vi "Get_Word_JSON.vi"(7 "API Key":string, 8 "error in (no error)":errorcluster, 10 "Word":string, 11 "client handle":T1) -> (0 "error out":errorcluster, 1 "Valid Definition?":bool, 2 "body":string, 3 "client handle out":T1)   [LabVIEW 2018, in "MerriamWebsterJSON.lvlib"]
uses:
  MerriamWebsterJSON.lvlib
  <vilib>/httpClient/ClientHandle.ctl
  <vilib>/httpClient/LabVIEWHTTPClient.lvlib
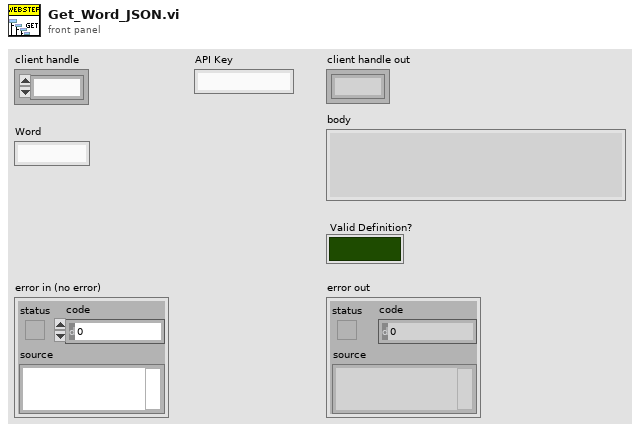
[diagram p1: front panel]
types:
  T1 = typedef "LabVIEWHTTPClient.lvlib/ClientHandle.ctl" = refnum<k1>
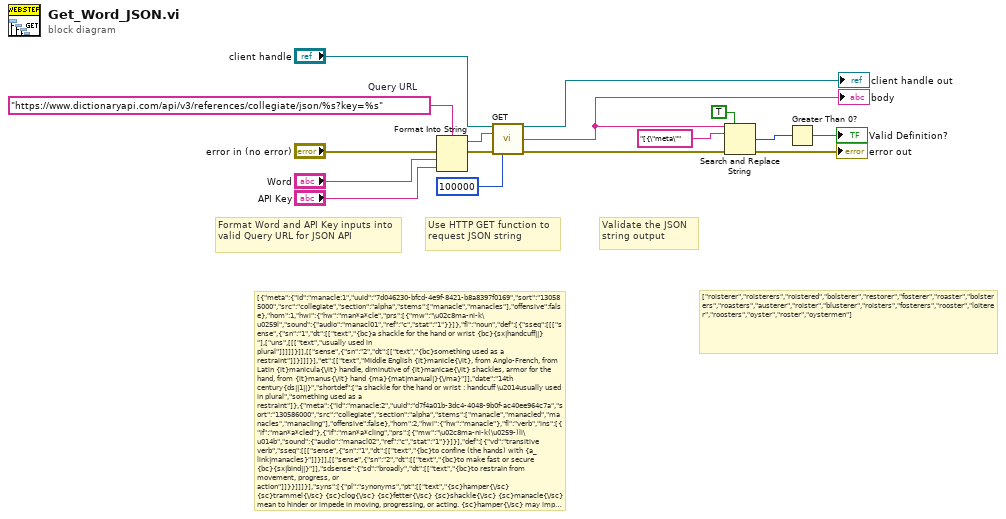
[diagram p0: block diagram]
diagram:
  w14 = "https://www.dictionaryapi.com/api/v3/references/collegiate/json/%s?key=%s"  # Query URL
  # "[{\"meta\":{\"id\":\"manacle:1\",\"uuid\":\"7d046230-bfcd-4e9f-8421-b8a8397f0169\",\"sort\":\"130585000\",\"src\":\"collegiate\",\"section\":\"alpha\",\"stems\":[\"manacle\",\"manacles\"],\"offensive\":false},\"hom\":1,\"hwi\":{\"hw\":\"man*a*cle\",\"prs\":[{\"mw\":\"\\u02c8ma-ni-k\\u0259l\",\"sound\":{\"audio\":\"manacl01\",\"ref\":\"c\",\"stat\":\"1\"}}]},\"fl\":\"noun\",\"def\":[{\"sseq\":[[[\"sense\",{\"sn\":\"1\",\"dt\":[[\"text\",\"{bc}a shackle for the hand or wrist {bc}{sx|handcuff||} \"],[\"uns\",[[[\"text\",\"usually used in plural\"]]]]]}]],[[\"sense\",{\"sn\":\"2\",\"dt\":[[\"text\",\"{bc}something used as a restraint\"]]}]]]}],\"et\":[[\"text\",\"Middle English {it}manicle{\\/it}, from Anglo-French, from Latin {it}manicula{\\/it} handle, diminutive of {it}manicae{\\/it} shackles, armor for the hand, from {it}manus{\\/it} hand {ma}{mat|manual|}{\\/ma}\"]],\"date\":\"14th century{ds||1||}\",\"shortdef\":[\"a shackle for the hand or wrist : handcuff \\u2014usually used in plural\",\"something used as a restraint\"]},{\"meta\":{\"id\":\"manacle:2\",\"uuid\":\"d7f4a01b-3dc4-4048-9b0f-ac40ee964c7a\",\"sort\":\"130586000\",\"src\":\"collegiate\",\"section\":\"alpha\",\"stems\":[\"manacle\",\"manacled\",\"manacles\",\"manacling\"],\"offensive\":false},\"hom\":2,\"hwi\":{\"hw\":\"manacle\"},\"fl\":\"verb\",\"ins\":[{\"if\":\"man*a*cled\"},{\"if\":\"man*a*cling\",\"prs\":[{\"mw\":\"\\u02c8ma-ni-k(\\u0259-)li\\u014b\",\"sound\":{\"audio\":\"manacl02\",\"ref\":\"c\",\"stat\":\"1\"}}]}],\"def\":[{\"vd\":\"transitive verb\",\"sseq\":[[[\"sense\",{\"sn\":\"1\",\"dt\":[[\"text\",\"{bc}to confine (the hands) with {a_link|manacles}\"]]}]],[[\"sense\",{\"sn\":\"2\",\"dt\":[[\"text\",\"{bc}to make fast or secure {bc}{sx|bind||}\"]],\"sdsense\":{\"sd\":\"broadly\",\"dt\":[[\"text\",\"{bc}to restrain from movement, progress, or action\"]]}}]]]}],\"syns\":[{\"pl\":\"synonyms\",\"pt\":[[\"text\",\"{sc}hamper{\\/sc} {sc}trammel{\\/sc} {sc}clog{\\/sc} {sc}fetter{\\/sc} {sc}shackle{\\/sc} {sc}manacle{\\/sc} mean to hinder or impede in moving, progressing, or acting. {sc}hamper{\\/sc} may imply the effect of any impeding or restraining influence. \"],[\"vis\",[{\"t\":\"{it}hampered{\\/it} the investigation by refusing to cooperate\"}]],[\"text\",\" {sc}trammel{\\/sc} suggests entangling by or confining within a net. \"],[\"vis\",[{\"t\":\"rules that {it}trammel{\\/it} the artist\\u0027s creativity\"}]],[\"text\",\" {sc}clog{\\/sc} usually implies a slowing by something extraneous or encumbering. \"],[\"vis\",[{\"t\":\"a court system {it}clogged{\\/it} by frivolous suits\"}]],[\"text\",\" {sc}fetter{\\/sc} suggests a restraining so severe that freedom to move or progress is almost lost. \"],[\"vis\",[{\"t\":\"a nation {it}fettered{\\/it} by an antiquated class system\"}]],[\"text\",\" {sc}shackle{\\/sc} and {sc}manacle{\\/sc} are stronger than {sc}fetter{\\/sc} and suggest total loss of freedom. \"],[\"vis\",[{\"t\":\"a mind {it}shackled{\\/it} by stubborn prejudice\"},{\"t\":\"a people {it}manacled{\\/it} by tyranny\"}]]]}],\"date\":\"14th century{ds||1||}\",\"shortdef\":[\"to confine (the hands) with manacles\",\"to make fast or secure : bind; broadly : to restrain from movement, progress, or action\"]}]"
  # "Validate the JSON string output"
  # "Use HTTP GET function to request JSON string"
  # "Format Word and API Key inputs into valid Query URL for JSON API"
  # "[\"roisterer\",\"roisterers\",\"roistered\",\"bolsterer\",\"restorer\",\"fosterer\",\"roaster\",\"bolsterers\",\"roasters\",\"austerer\",\"roister\",\"blusterer\",\"roisters\",\"fosterers\",\"rooster\",\"loiterer\",\"roosters\",\"oyster\",\"roster\",\"oystermen\"]"
  n1 = Format Into String(format string=w14, error in="error in (no error)", "Word", "API Key") -> (resulting string=w9:string, error out=w10:errorcluster)  [unwired: 1 in]
  n2 = call <vilib>:"GET.vi"("client handle"="client handle", "url"=w9, "error in (no error)"=w10, "timeout (10000)"=100000) -> ("client handle out"=→"client handle out":T1, "body"=w1:string, "error out"=w5:errorcluster)  [unwired: 8 in, 1 out]
  "body" <- w1
  n3 = Search and Replace String(replace all?=TRUE ("replace all? (F)"), input string=w1, search string="[{\"meta\"", error in=w5) -> (number of replacements=w3:i32, error out=→"error out":errorcluster)  [unwired: 4 in, 2 out]
  n4 = Greater Than 0?(x=w3) -> (x > 0?=→"Valid Definition?":bool)
